vi "CreateTimestampedLogfile.vi"(9 "Timestamp":timestamp, 10 "Name":string, 11 "Path":path) -> (0 "error out":errorcluster, 3 "Byte Stream File out":refnum<file>)   [LabVIEW 2011]
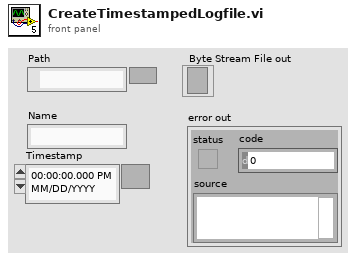
[diagram p1: front panel]
types:
  T1 = enum16{"open", "replace", "create", "open or create", "replace or create", "replace or create with confirmation"}
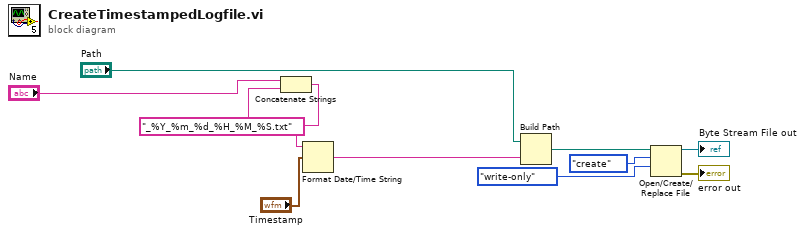
[diagram p0: block diagram]
diagram:
  n1 = Concatenate Strings("Name", "_%Y_%m_%d_%H_%M_%S.txt" ("time format string (%c)")) -> (w11:string)
  n2 = Format Date/Time String(time format string (%c)=w11, seconds (now)="Timestamp") -> (date/time string=w4:string)  [unwired: 1 in]
  n3 = Build Path(base path="Path", name or relative path=w4) -> (appended path=w5:path)
  n4 = Open/Create/Replace File(file path (use dialog)=w5, operation (0:open)=T1."create", access (0:read/write)=enum16{"read/write", "read-only", "write-only"}."write-only") -> (refnum out=→"Byte Stream File out":refnum<file>, error out=→"error out":errorcluster)  [unwired: 3 in, 1 out]
